vi "Hindbrain Main.vi"(10 "Boat Type":T4(ring)=enum."Damn Yankee", 11 "NotifierReff":T5) -> ()   [LabVIEW 2013]
doc: "Place to hold all the hindbrain code."
uses:
  Data/TypeDefs/Notifiers.ctl
  Data/TypeDefs/UTM Location.ctl
  Data/TypeDefs/Sail Set Suggestions.ctl
  Data/TypeDefs/Rudder Set Suggestions.ctl
  Data/TypeDefs/OverrideInformation.ctl
  Data/TypeDefs/OverrideMode.ctl
  Data/TypeDefs/MotorSetup.ctl
  Data/TypeDefs/DynamixelSetupInfo.ctl
  Data/TypeDefs/AirmarStatus.ctl
  Data/TypeDefs/HardwareOnline.ctl
  Data/TypeDefs/GPS-Compass Queue Cluster.ctl
  Data/TypeDefs/WindData Queue Cluster.ctl
  <vilib>/myRIO/Common/Instrument Driver Framework/myRIO v1.0/UART/vis/myRIO v1.0 Close UART.vi
  <vilib>/myRIO/Common/Instrument Driver Framework/Utilities/vis/FPGA Ref Manager.vi
  <vilib>/myRIO/Common/Instrument Driver Framework/myRIO v1.0/myRIO v1.0 Reset FPGA.vi
  <vilib>/myRIO/Instrument Drivers/Utilities/Utilities.lvlib
panel:
  in  "output cluster":T3
  in  "Wind Direction":dbl
  in  "Wind Speed":dbl
  out "Replace? (<6?)":bool
  out "Battery Volts":dbl
  out "UDP Time Out?":bool
  out "String received from XBee":string
  out "String written to XBee":string
  in  "XBee Serial Port":refnum<visa-resource-name>="LPT1"
  in  "Queue timeout (ms)":i32=50
  # "Little boat"
  # "XBee"
  # "If you're getting no strings, do you have the right COM port?"
  # "Camera"
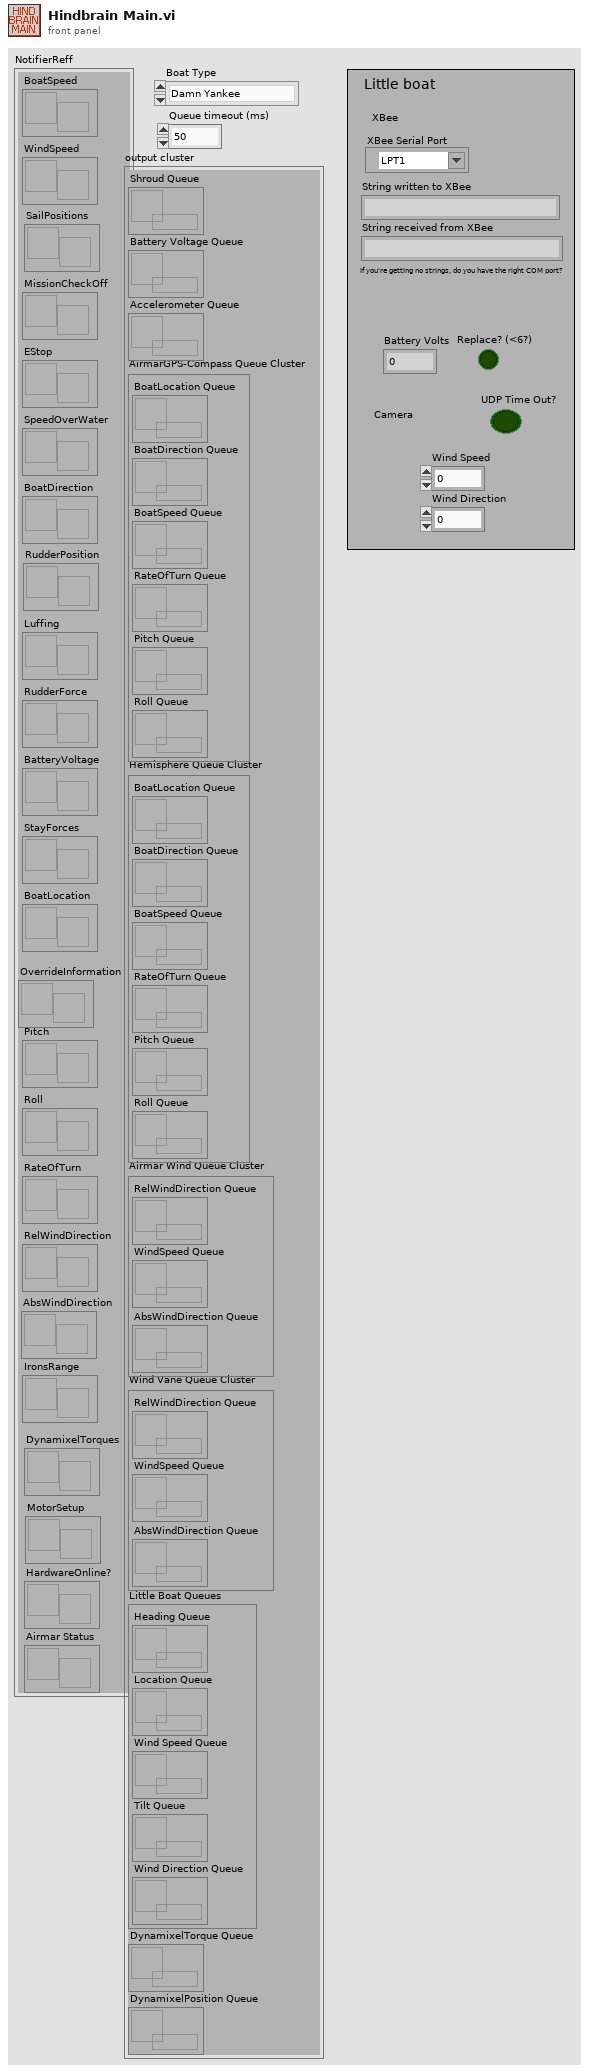
[diagram p1: front panel]
types:
  T1 = typedef "GPS-Compass Queue Cluster.ctl" = cluster{"BoatLocation Queue":refnum<queue>, "BoatDirection Queue":refnum<queue>, "BoatSpeed Queue":refnum<queue>, "RateOfTurn Queue":refnum<queue>, "Pitch Queue":refnum<queue>, "Roll Queue":refnum<queue>}
  T2 = typedef "WindData Queue Cluster.ctl" = cluster{"RelWindDirection Queue":refnum<queue>, "WindSpeed Queue":refnum<queue>, "AbsWindDirection Queue":refnum<queue>}
  T3 = cluster{"Shroud Queue":refnum<queue>, "Battery Voltage Queue":refnum<queue>, "Accelerometer Queue":refnum<queue>, "AirmarGPS-Compass Queue Cluster":T1, "Hemisphere Queue Cluster":T1, "Airmar Wind Queue Cluster":T2, "Wind Vane Queue Cluster":T2, "Little Boat Queues":cluster{"Heading Queue":refnum<queue>, "Location Queue":refnum<queue>, "Wind Speed Queue":refnum<queue>, "Tilt Queue":refnum<queue>, "Wind Direction Queue":refnum<queue>}, "DynamixelTorque Queue":refnum<queue>, "DynamixelPosition Queue":refnum<queue>}
  T4 = enum16{"Blackbody Radiation", "Little boats", "Simulation", "Damn Yankee"}
  T5 = typedef "Notifiers.ctl" = cluster{"BoatSpeed":refnum<notifier>, "WindSpeed":refnum<notifier>, "MissionCheckOff":refnum<notifier>, "EStop":refnum<notifier>, "SpeedOverWater":refnum<notifier>, "BoatDirection":refnum<notifier>, "Luffing":refnum<notifier>, "RudderForce":refnum<notifier>, "BatteryVoltage":refnum<notifier>, "StayForces":refnum<notifier>, "BoatLocation":refnum<notifier>, "Pitch":refnum<notifier>, "Roll":refnum<notifier>, "RateOfTurn":refnum<notifier>, "RelWindDirection":refnum<notifier>, "SailPositions":refnum<notifier>, "RudderPosition":refnum<notifier>, "IronsRange":refnum<notifier>, "AbsWindDirection":refnum<notifier>, "OverrideInformation":refnum<notifier>, "DynamixelTorques":refnum<notifier>, "MotorSetup":refnum<notifier>, "Airmar Status":refnum<notifier>, "HardwareOnline?":refnum<notifier>}
  T6 = typedef "PWM.lvlib/PWM Reference.ctl" = cluster{"myRIO Reference":T7, "PWM Channels Enum":T11, "PWM Configuration":T12}
  T7 = typedef "myRIO Generic Hardware Reference.ctl" = cluster{"myRIO Model":T8, "myRIO Hardware Reference":T9}
  T8 = typedef "Hardware Version Enum.ctl" = enum16{"Unknown", "myRIO-1900", "myRIO-1950"}
  T9 = typedef "myRIO v1.0 Reference.ctl" = cluster{"Generic FPGA Reference":T10, "Allow multiple opens":bool}
  T10 = typedef "Generic FPGA Reference.ctl" = refnum<k20>
  T11 = typedef "PWM Channels Enum.ctl" = enum16{"Not Connected", "C/PWM0", "C/PWM1", "A/PWM0", "A/PWM1", "A/PWM2", "B/PWM0", "B/PWM1", "B/PWM2"}
  T12 = typedef "PWM.lvlib/PWM Configuration.ctl" = cluster{"Frequency":dbl, "Duty Cycle":dbl}
  T13 = cluster{"Airmar VISA Resource":refnum<visa-resource-name>, "Hemisphere VISA Resource":refnum<visa-resource-name>, "Dynamixel VISA Resource":refnum<visa-resource-name>, "Airmar Error":errorcluster, "Hemisphere Error":errorcluster, "Dynamixel Error":errorcluster, "OLD Airmar Refernce Number":refnum<visa-resource-name>, "Rudder PWM Ref":T6, "Rudder Error":errorcluster}
  T14 = cluster{"Heading Queue":refnum<queue>, "Location Queue":refnum<queue>, "Wind Speed Queue":refnum<queue>, "Tilt Queue":refnum<queue>, "Wind Direction Queue":refnum<queue>}
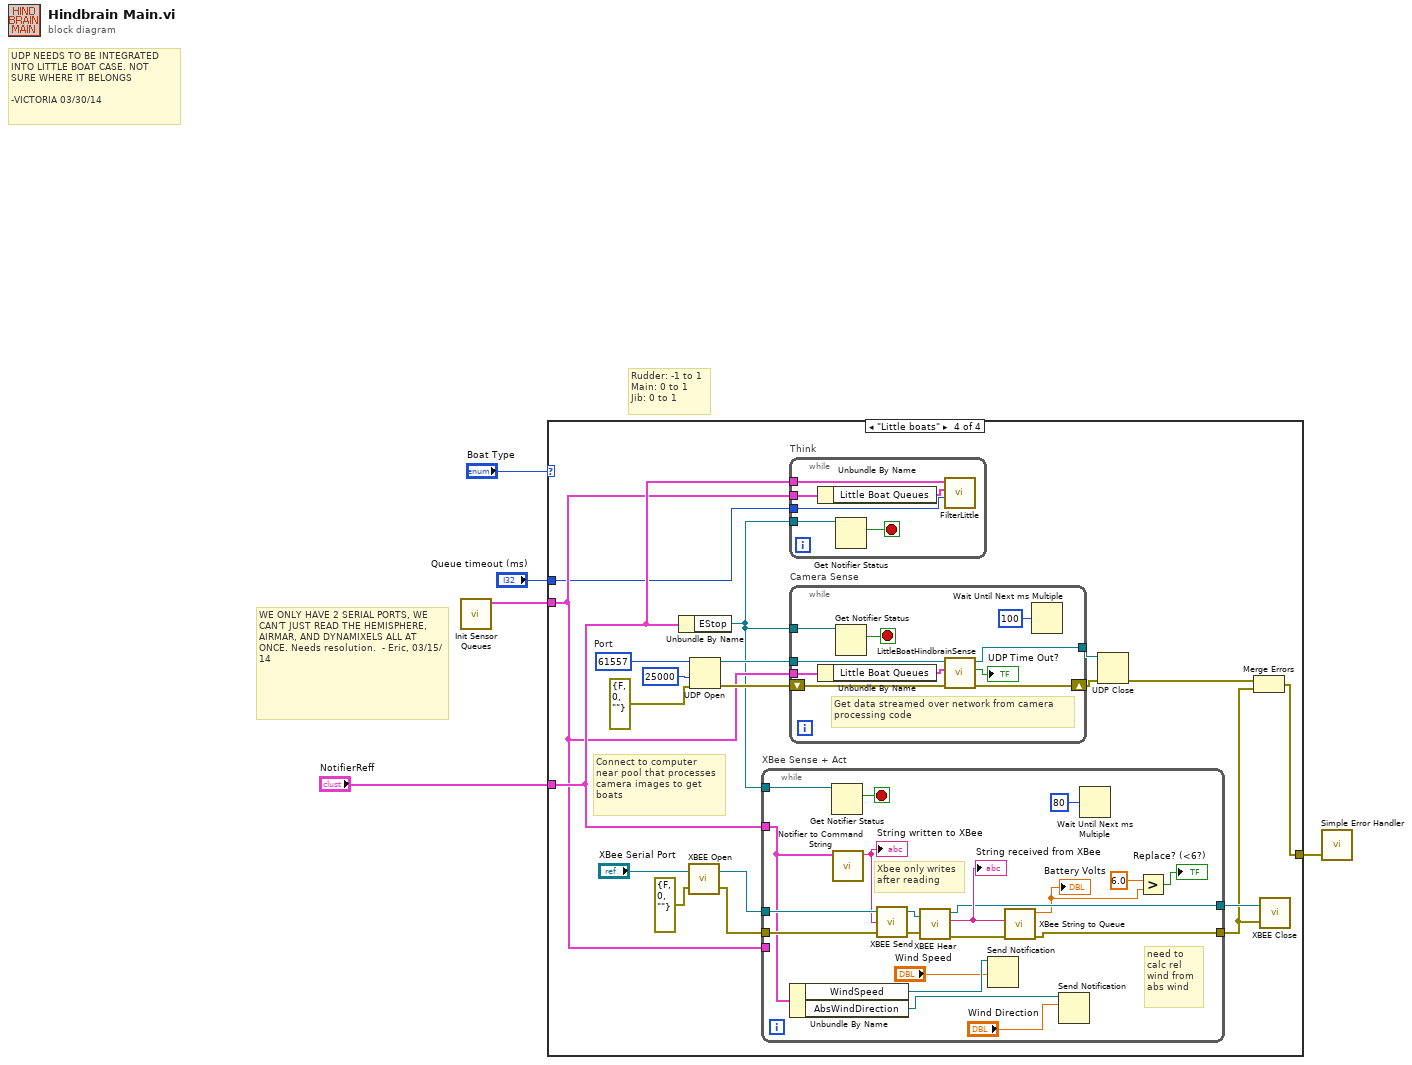
[diagram p0: block diagram]
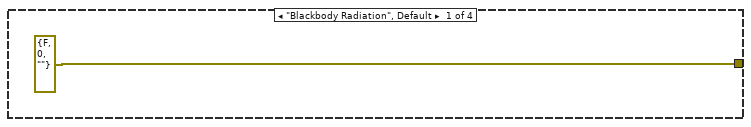
[diagram p2: hidden frame]
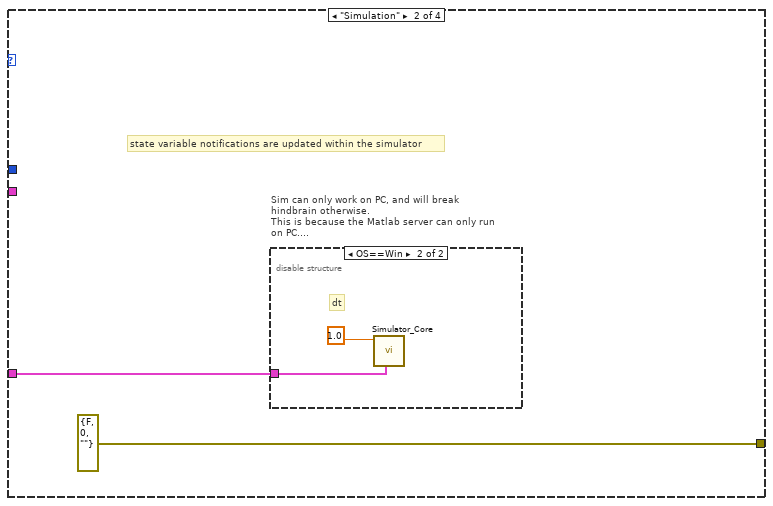
[diagram p3: hidden frame]
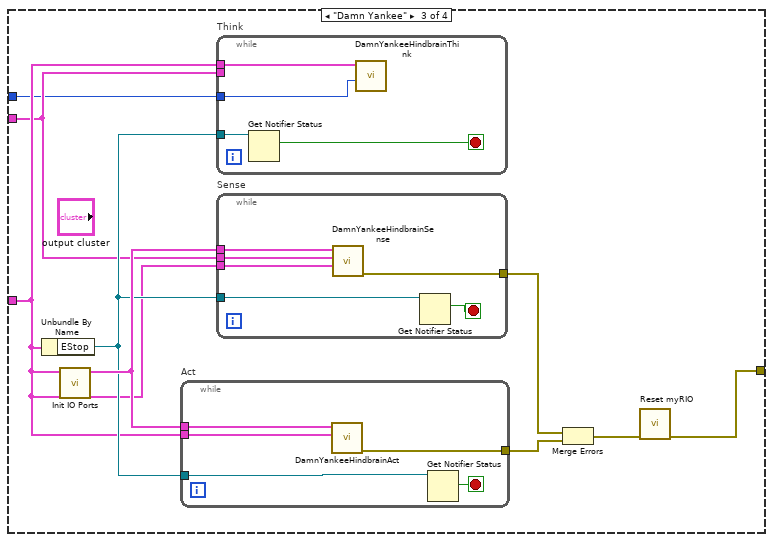
[diagram p5: hidden frame]
diagram:
  # "Rudder: -1 to 1\nMain: 0 to 1 \nJib: 0 to 1"
  # "UDP NEEDS TO BE INTEGRATED\nINTO LITTLE BOAT CASE. NOT \nSURE WHERE IT BELONGS\n\n-VICTORIA 03/30/14"
  # "WE ONLY HAVE 2 SERIAL PORTS, WE CAN'T JUST READ THE HEMISPHERE, AIRMAR, AND DYNAMIXELS ALL AT ONCE. Needs resolution.  - Eric, 03/15/14"
  n1 = call "Init Sensor Queues.vi"() -> ("output cluster"=w5:T3)  [unwired: 11 in]
  n2 = case shown="\"Little boats\"" "Boat Type" {
    tunnel: w5 -> [_ _ w12 w42]
    tunnel: "NotifierReff" -> [_ w8 w13 w46]
    tunnel: [errorcluster {"status"=FALSE, "code"=0, "source"=""} ("error IO") errorcluster {"status"=FALSE, "code"=0, "source"=""} ("error IO") w15 w53] -> w4
    tunnel: "Queue timeout (ms)" -> [_ _ w11 w35]
    frame "Blackbody Radiation", Default {
    }
    frame "Simulation" {
      # "state variable notifications are updated within the simulator"
      n3 = disable-structure "Sim can only work on PC, and will break hindbrain otherwise.\nThis is because the Matlab server can only run on PC.\nTherefore, we have to actually disable (not just case structure)\nthe simulator when not on PC." shown="OS==Win" {
        disable-tunnel: w8 -> [_ w9]
        frame condition #0 {
        }
        frame condition #1 (active) {
          # "dt"
          n4 = call "Simulator_Core.vi"("NotifierReff"=w9, "dt"=1.0) -> ()  [unwired: 10 in]
        }
      }
    }
    frame "Damn Yankee" {
      n5 = Unbundle By Name(w13) -> ("EStop"=w14:refnum<notifier>)
      n6 = call "Init IO Ports.vi"("NotifierReff"=w13) -> ("IO Port Cluster"=w19:T13)  [unwired: 10 in]
      n7 = while "Act" {
        tunnel: w19 -> [w34]
        tunnel: w13 -> [w33]
        tunnel: [w32] -> w17
        tunnel: w14 -> [w30]
        stop <- w31 stop-if-true
        n8 = call "DamnYankeeHindbrainAct.vi"("NotifierReff"=w33, "IO Port Cluster"=w34) -> ("error out"=w32:errorcluster)  [unwired: 9 in]
        n9 = Get Notifier Status(notifier=w30) -> (current notification=w31:bool)  [unwired: 1 in, 4 out]
      }
      n10 = while "Think" {
        tunnel: w14 -> [w23]
        tunnel: w12 -> [_]
        tunnel: w13 -> [w21]
        tunnel: w11 -> [w20]
        stop <- w22 stop-if-true
        n11 = Get Notifier Status(notifier=w23) -> (current notification=w22:bool)  [unwired: 1 in, 4 out]
        n12 = call "DamnYankeeHindbrainThink.vi"("Queue timeout (ms)"=w20, "Notifier References"=w21) -> ()  [unwired: 10 in]
      }
      n13 = while "Sense" {
        tunnel: w19 -> [w29]
        tunnel: w13 -> [w28]
        tunnel: w12 -> [w24]
        tunnel: [w27] -> w18
        tunnel: w14 -> [w26]
        stop <- w25 stop-if-true
        n14 = call "DamnYankeeHindbrainSense.vi"("Notifier References"=w28, "Data Queue clusters"=w24, "IO Port Cluster"=w29) -> ("error out"=w27:errorcluster)  [unwired: 8 in]
        n15 = Get Notifier Status(notifier=w26) -> (current notification=w25:bool)  [unwired: 1 in, 4 out]
      }
      n16 = Merge Errors "Merge Errors"(w18, w17) -> (w16:errorcluster)
      n17 = call <vilib>:"Reset myRIO.vi"("error in (no error)"=w16) -> ("error out"=w15:errorcluster)  [unwired: 10 in]
    }
    frame "Little boats" {
      w51 = u16 61557  # Port
      # "Connect to computer\nnear pool that processes\ncamera images to get\nboats"
      n18 = Unbundle By Name(w46) -> ("EStop"=w36:refnum<notifier>)
      n19 = call "XBEE Open.vi"("error in"=errorcluster {"status"=FALSE, "code"=0, "source"=""}, "VISA resource name"="XBee Serial Port") -> ("error out"=w45:errorcluster, "VISA resource name out"=w47:refnum<visa-resource-name>)
      n20 = UDP Open(8:errorcluster {"status"=FALSE, "code"=0, "source"=""} ("error in (no error)"), 9:25000 ("timeout ms (25000)"), 11:w51) -> (port=w44:refnum<k16>, 0:w43:errorcluster)  [unwired: 2 in, 1 out]
      n21 = while "XBee Sense + Act" {
        tunnel: w47 -> [w82]
        tunnel: w46 -> [w68]
        tunnel: w36 -> [w83]
        tunnel: w42 -> [_]
        tunnel: [w73] -> w41
        tunnel: w45 -> [w81]
        tunnel: [w72] -> w40
        stop <- w77 stop-if-true
        # "Xbee only writes\nafter reading"
        # "need to\ncalc rel\nwind from\nabs wind"
        n22 = Unbundle By Name(w68) -> ("WindSpeed"=w66:refnum<notifier>, "AbsWindDirection"=w67:refnum<notifier>)
        n23 = Get Notifier Status(notifier=w83) -> (current notification=w77:bool)  [unwired: 1 in, 4 out]
        n24 = call "Notifier to Command String.vi"("NotifierReff"=w68) -> ("String"=w80:string)  [unwired: 10 in]
        "String written to XBee" <- w80
        n25 = call "XBEE Send.vi"("error in (no error)"=w81, "String"=w80, "VISA resource name"=w82) -> ("error out"=w78:errorcluster, "VISA resource name out"=w79:refnum<visa-resource-name>)  [unwired: 1 out]
        n26 = call "XBEE Hear.vi"("VISA resource name"=w79, "error in (no error)"=w78) -> ("VISA resource name out"=w73:refnum<visa-resource-name>, "String Received"=w76:string, "error out"=w75:errorcluster)  [unwired: 1 out]
        "String received from XBee" <- w76
        n27 = Send Notification(notification="Wind Speed", notifier=w66) -> ()  [unwired: 1 in, 2 out]
        n28 = call "XBee String to Queue.vi"("error in (no error)"=w75, "String Received"=w76) -> ("error out"=w72:errorcluster, "Battery Volts"=w71:dbl)  [unwired: 8 in]
        "Battery Volts" <- w71
        n29 = Send Notification(notification="Wind Direction", notifier=w67) -> ()  [unwired: 1 in, 2 out]
        n30 = Wait Until Next ms Multiple(millisecond multiple=u32 80) -> ()  [unwired: 1 out]
        n31 = Greater?(x=6.0, y=w71) -> (0:→"Replace? (<6?)":bool)
      }
      n32 = while "Think" {
        tunnel: w36 -> [w89]
        tunnel: w42 -> [w87]
        tunnel: w46 -> [w85]
        tunnel: w35 -> [w84]
        stop <- w88 stop-if-true
        n33 = Unbundle By Name(w87) -> ("Little Boat Queues"=w86:T14)
        n34 = Get Notifier Status(notifier=w89) -> (current notification=w88:bool)  [unwired: 1 in, 4 out]
        n35 = call "FilterLittle.vi"("timeout in ms"=w84, "Little Boat Queues"=w86, "NotifierReff"=w85) -> ()  [unwired: 9 in]
      }
      n36 = while "Camera Sense" {
        tunnel: w44 -> [w62]
        tunnel: w42 -> [w61]
        tunnel: [w59] -> w39
        tunnel: w36 -> [w56]
        shift-right: [w58] -> w38
        shift-left: w43 -> [w63]
        stop <- w55 stop-if-true
        # "Get data streamed over network from camera\nprocessing code"
        n37 = Unbundle By Name(w61) -> ("Little Boat Queues"=w60:T14)
        n38 = Get Notifier Status(notifier=w56) -> (current notification=w55:bool)  [unwired: 1 in, 4 out]
        n39 = call "LittleBoatHindbrainSense.vi"("error in (no error)"=w63, "Little Boat Queues"=w60, "connection ID"=w62) -> ("error out"=w58:errorcluster, "UDP Time Out?"=→"UDP Time Out?":bool, "connection ID out"=w59:refnum<k16>)  [unwired: 6 in]
        n40 = Wait Until Next ms Multiple(millisecond multiple=u32 100) -> ()  [unwired: 1 out]
      }
      n41 = UDP Close(connection ID=w39, 8:w38) -> (error out=w37:errorcluster)  [unwired: 1 out]
      n42 = Merge Errors "Merge Errors"(w37, w40) -> (w53:errorcluster)
      n43 = call "XBEE Close.vi"("error in (no error)"=w40, "VISA resource name"=w41) -> ()
    }
  }
  n44 = call <vilib>:"Simple Error Handler.vi"("error in (no error)"=w4) -> ()  [unwired: 4 in, 5 out]
